vi "ngi get dataset secure.vi"(0 "ID":u16, 1 "Downloaded dataset":T4(array[cluster]), 3 "num sensor":i32[](array[numeric]), 4 "last packet type":u8[](array[numeric]), 5 "error in (no error)":errorcluster, 6 "State":u16(ring) items=["Init array", "Send get", "recive data", "abort secure download"], 7 "Node":i32=1, 8 "max download atempts":u8=10, 9 "download timeout":dbl=60.0 format="%#_13g", 10 "event_datadir":string, 12 "Recent events 2":T1(array[cluster]) {"SPS" format="%.1f"}, 13 "mac adresses":T3) -> (15 "Dataset":waveform(dbl)[][](array[waveform]), 16 "is downloading":bool[](array[boolean]), 18 "Safe Download":T2(array[cluster]), 19 "error out":errorcluster)   [LabVIEW 2017]
panel:
  out "busy?":bool[](array[boolean])
  out "channel mask":u8
  out "current time":timestamp
  out "dataset is complet":bool
  out "inserting data into array":bool
  out "last downloaded sample":u32
  out "num downloaded samples":u32
  out "dataset transfer completed":bool
  out "num samples in packet":i32
  out "Array":i32[][][](array[numeric])
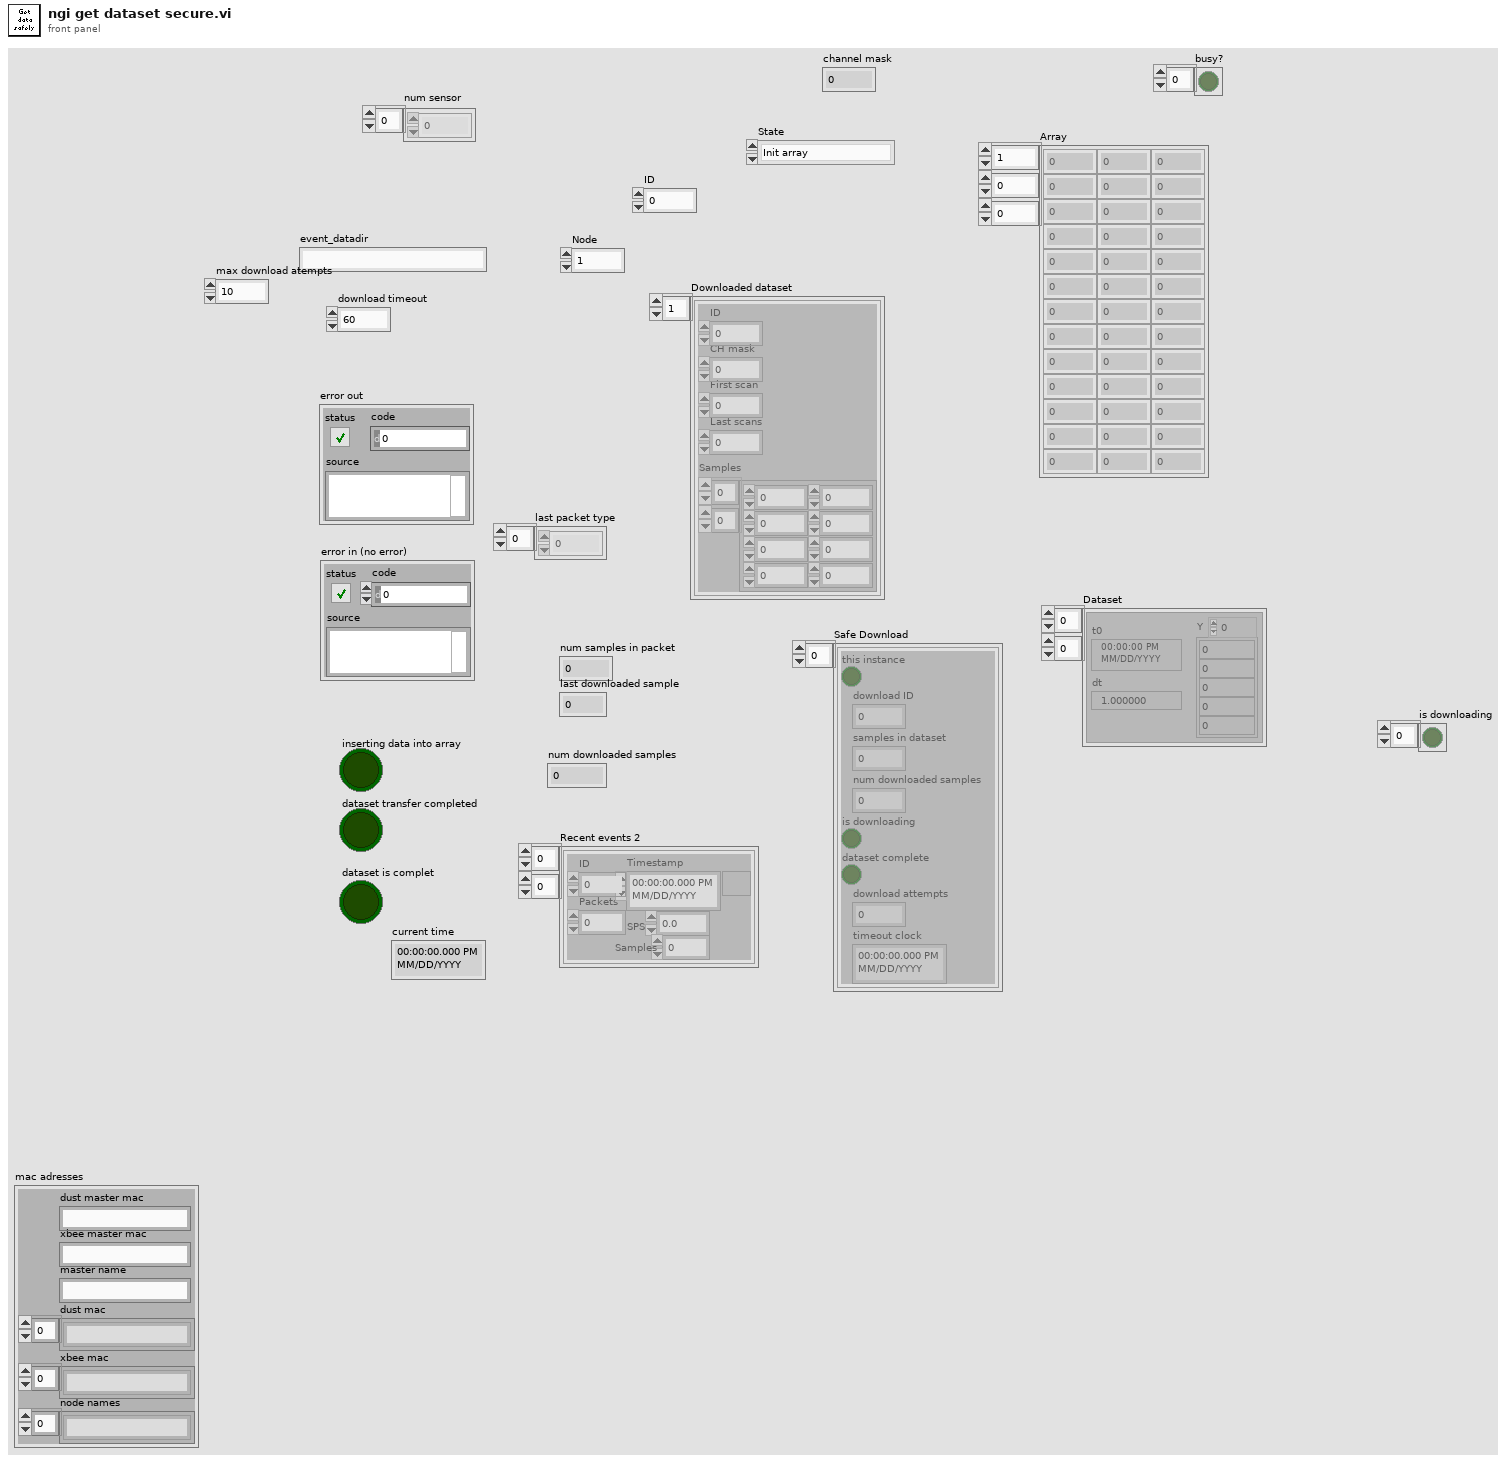
[diagram p1: front panel]
types:
  T1 = cluster{"ID":u16, "Timestamp":timestamp, "Packets":u16, "SPS":dbl, "Samples":u16}[][]
  T2 = cluster{"this instance":bool, "download ID":u32, "samples in dataset":u32, "num downloaded samples":u32, "is downloading":bool, "dataset complete":bool, "download attempts":u32, "timeout clock":timestamp}[]
  T3 = cluster{"dust master mac":string, "xbee master mac":string, "master name":string, "dust mac":string[], "xbee mac":string[], "node names":string[]}
  T4 = cluster{"ID":u16, "CH mask":u8, "First scan":u32, "Last scans":u32, "Samples":i32[][]}[]
  T5 = cluster{"this instance":bool, "download ID":u16, "samples in dataset":u32, "num downloaded samples":u32, "is downloading":bool, "dataset complete":bool, "download attempts":u32, "timeout clock":timestamp}
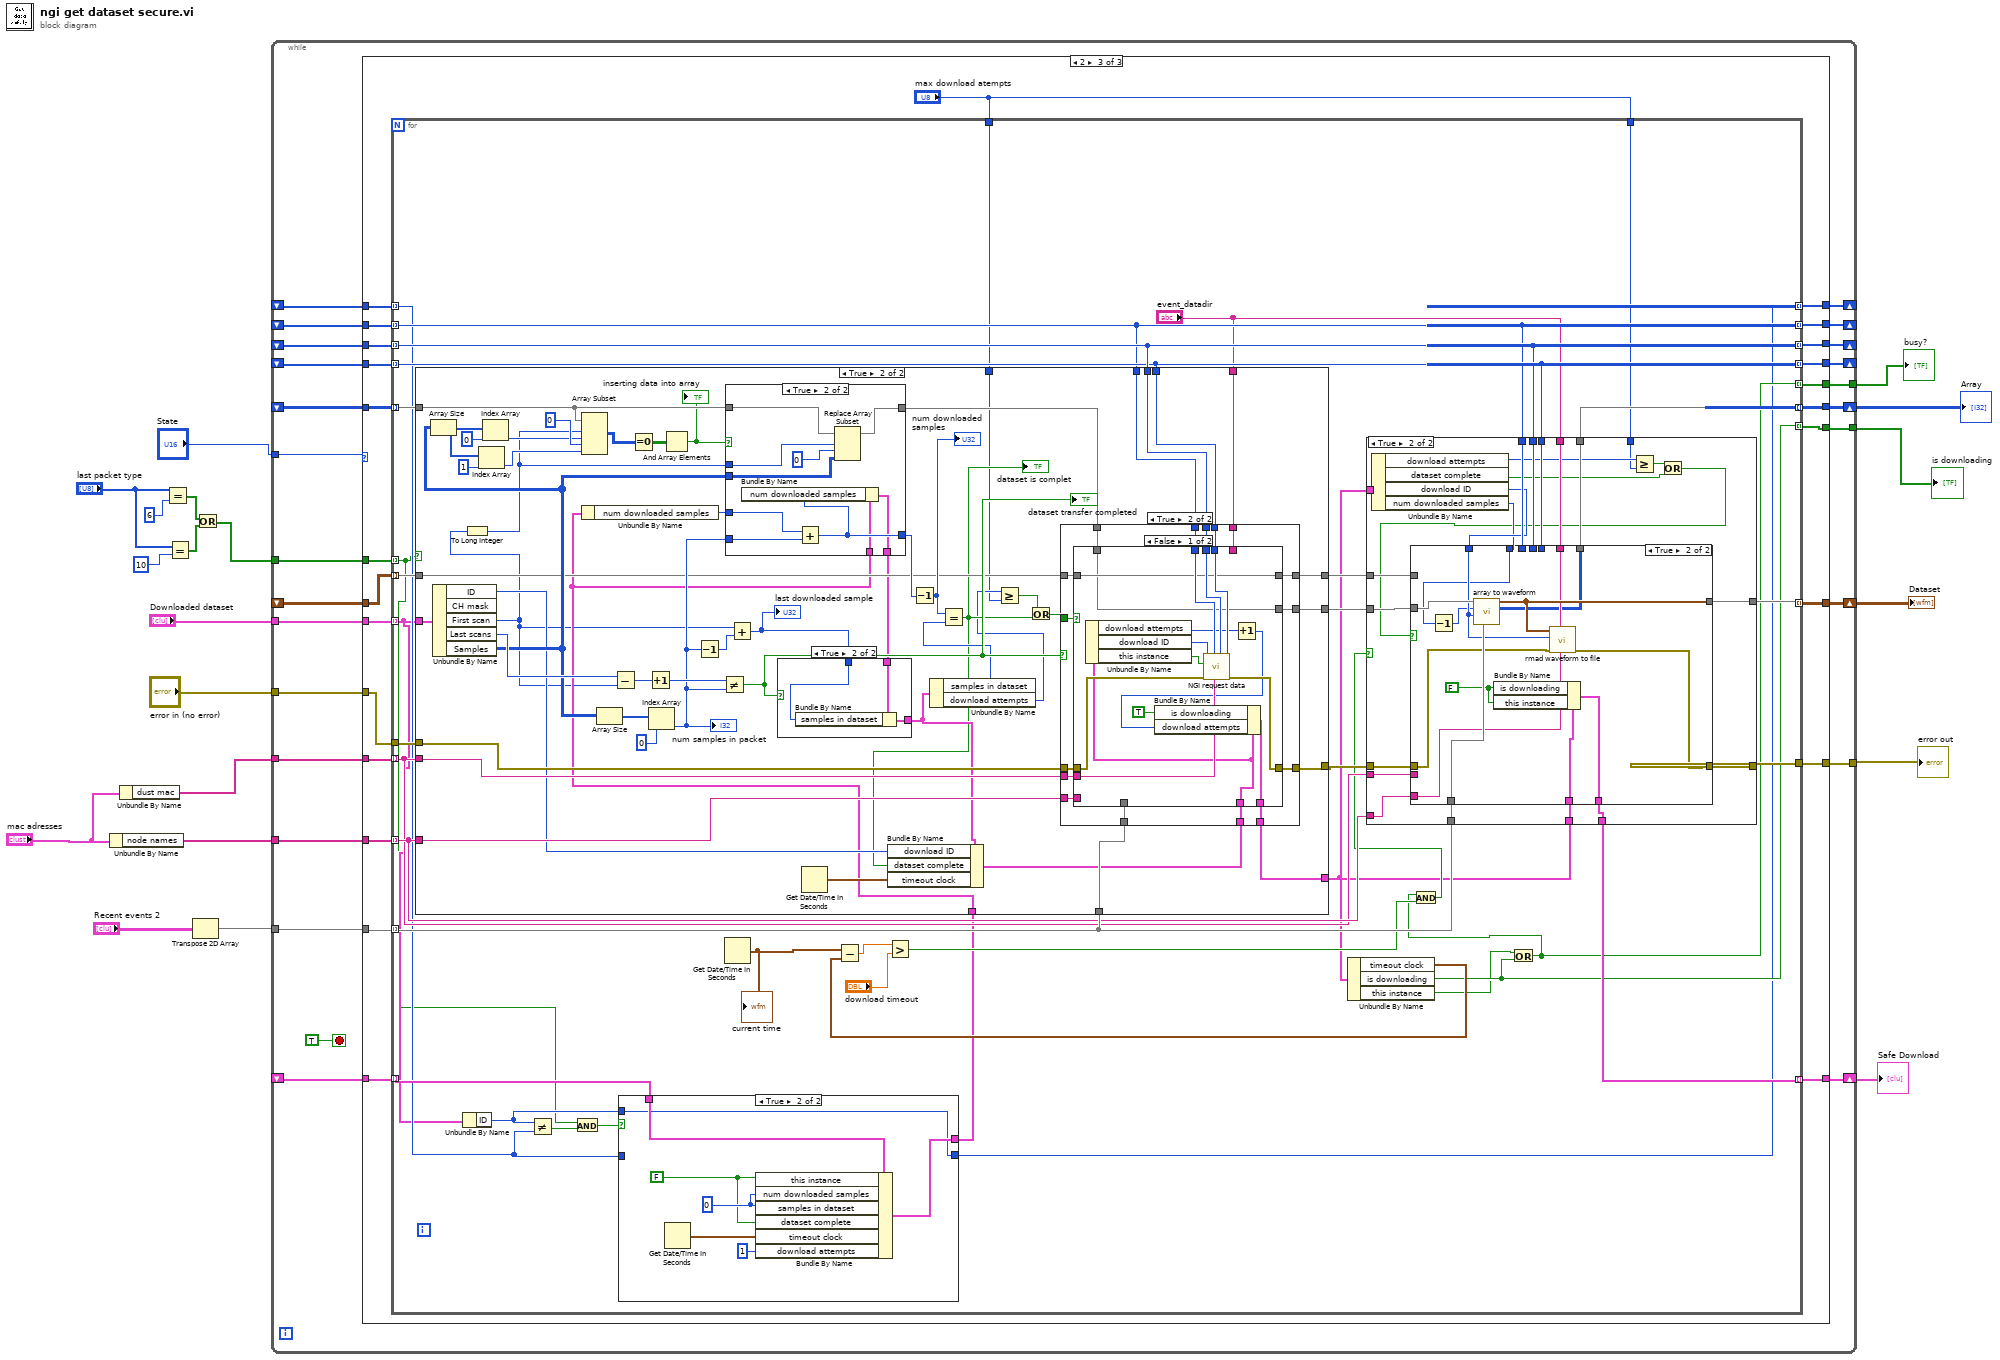
[diagram p0: block diagram]
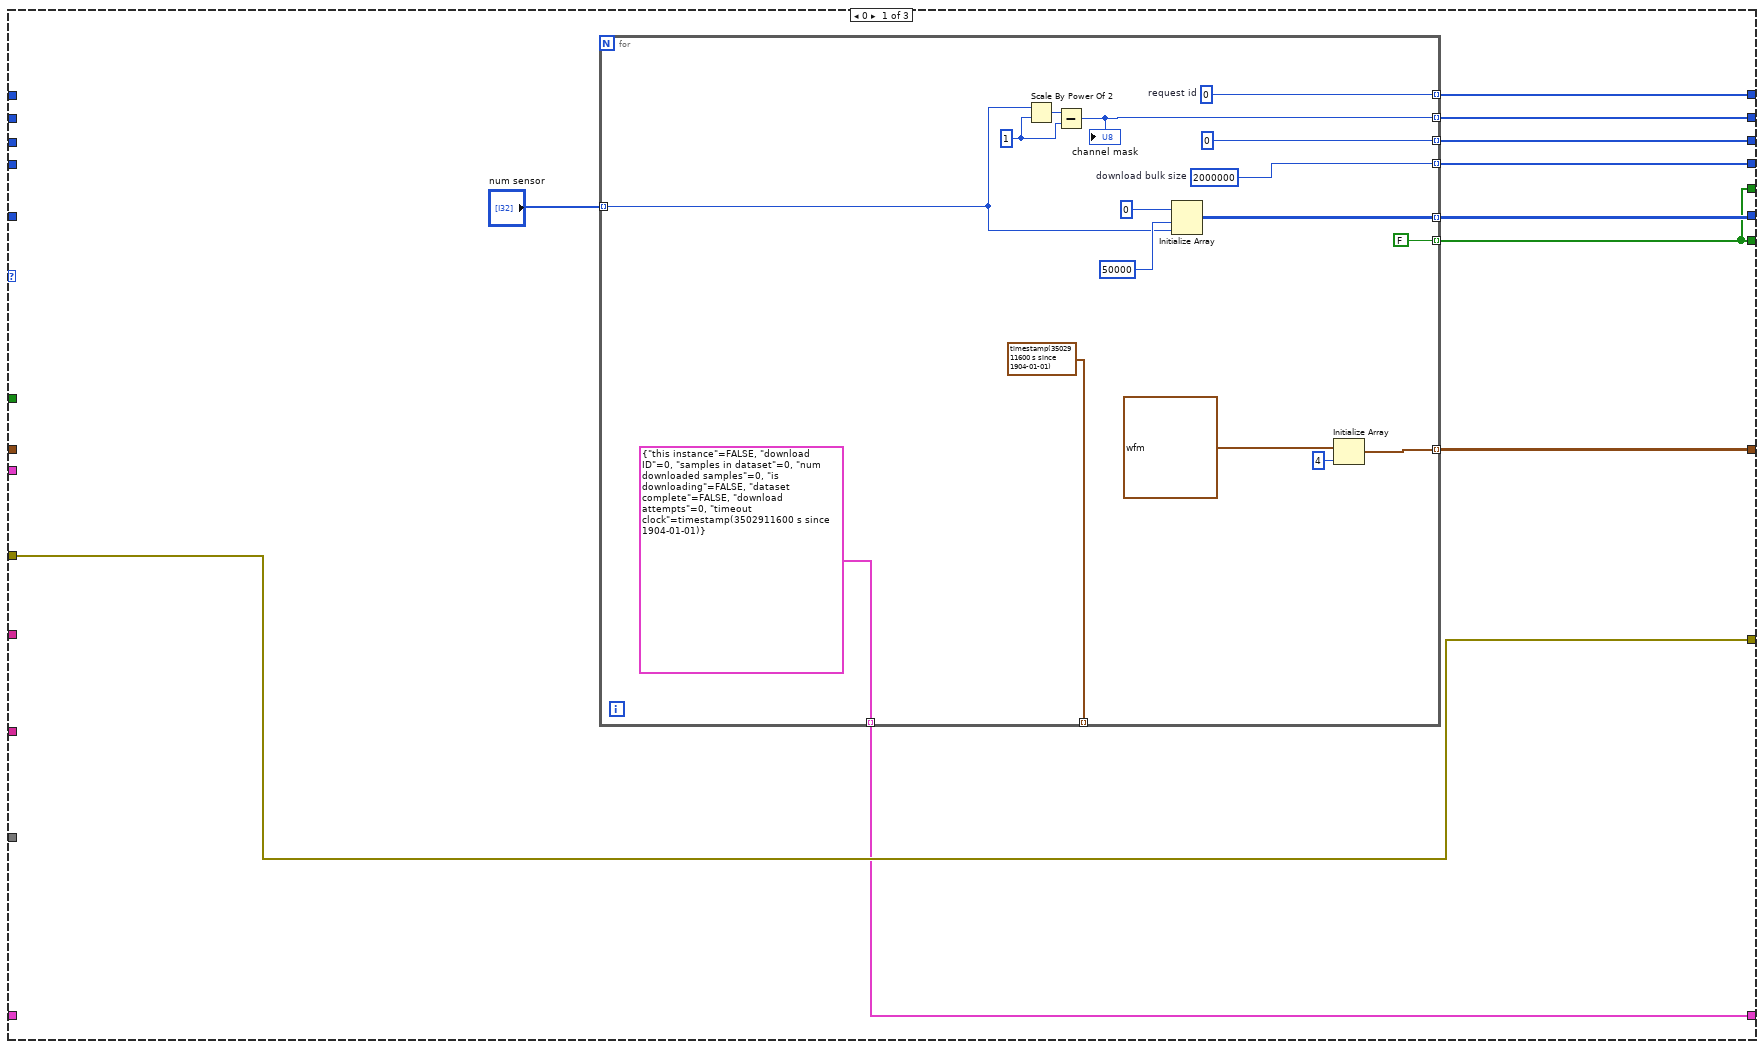
[diagram p2: hidden frame]
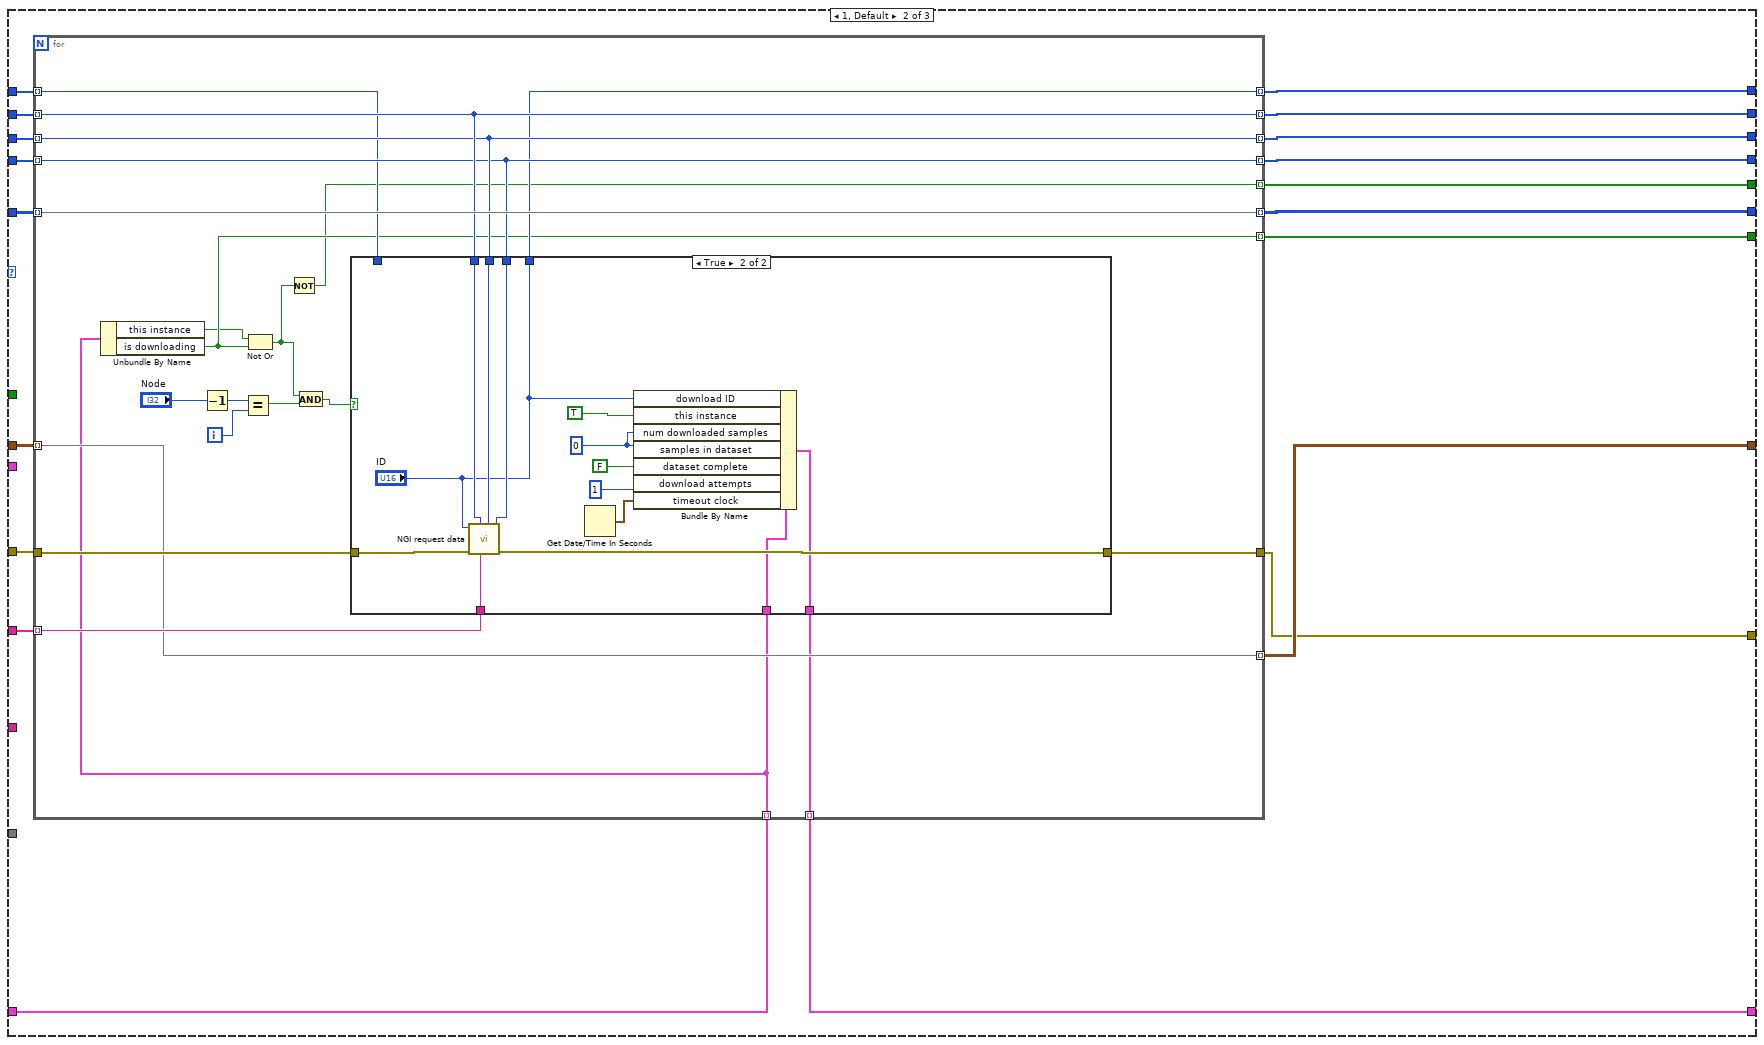
[diagram p3: hidden frame]
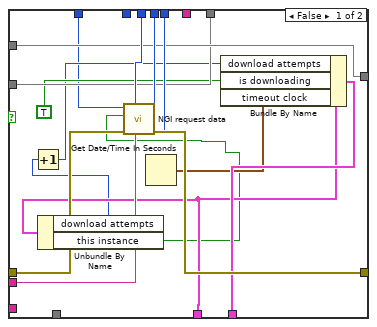
[diagram p7: hidden frame]
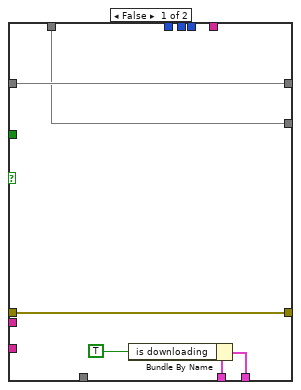
[diagram p9: hidden frame]
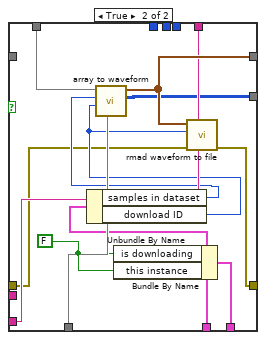
[diagram p10: hidden frame]
diagram:
  n1 = Unbundle By Name("mac adresses") -> ("node names"=w14:string[])
  n2 = Unbundle By Name("mac adresses") -> ("dust mac"=w11:string[])
  n3 = Equal?(x="last packet type", y=u8 6) -> (x = y?=w2:bool[])
  n4 = Equal?(x="last packet type", y=u8 10) -> (x = y?=w3:bool[])
  n5 = Transpose 2D Array(2D array="Recent events 2") -> (transposed array=w15:T1)
  n6 = Or(x=w2, y=w3) -> (x .or. y?=w1:bool[])
  n7 = while {
    tunnel: [w44] -> w10
    tunnel: "error in (no error)" -> [w43]
    tunnel: "State" -> [w31]
    tunnel: "Downloaded dataset" -> [w42]
    shift-right: [w25] -> w17
    shift-left: _ -> [w37]
    shift-right: [w38] -> _
    shift-left: _ -> [w33]
    shift-right: [w39] -> _
    shift-left: _ -> [w34]
    shift-right: [w40] -> _
    shift-left: _ -> [w35]
    shift-right: [w41] -> _
    shift-left: _ -> [w36]
    tunnel: w1 -> [w32]
    tunnel: w11 -> [w30]
    tunnel: w15 -> [w29]
    tunnel: w14 -> [w28]
    shift-right: [w27] -> w13
    shift-left: _ -> [w26]
    shift-right: [w24] -> w9
    shift-left: _ -> [w23]
    tunnel: [w22] -> w8
    tunnel: [w21] -> w6
    stop <- TRUE stop-if-true
    n8 = case shown="2" w31 {
      tunnel: [w49 w76 w134] -> w44
      tunnel: w43 -> [w49 w90 w141]
      tunnel: w42 -> [_ _ w152]
      tunnel: [w55 w81 w150] -> w25
      tunnel: [w54 w83 w143] -> w41
      tunnel: [w53 w85 w145] -> w40
      tunnel: [w52 w87 w147] -> w39
      tunnel: [w51 w89 w149] -> w38
      tunnel: w37 -> [_ w80 w151]
      tunnel: w36 -> [_ w82 w142]
      tunnel: w35 -> [_ w84 w144]
      tunnel: w34 -> [_ w86 w146]
      tunnel: w33 -> [_ w88 w148]
      tunnel: w32 -> [_ _ w140]
      tunnel: w30 -> [_ w79 w139]
      tunnel: w29 -> [_ _ w138]
      tunnel: w28 -> [_ _ w137]
      tunnel: [w50 w77 w135] -> w27
      tunnel: w26 -> [_ w78 w136]
      tunnel: [w48 w74 w132] -> w24
      tunnel: w23 -> [_ w75 w133]
      tunnel: [w46 w73 w131] -> w22
      tunnel: [w46 w72 w130] -> w21
      frame 0 {
        n9 = for {
          tunnel: [w70] -> w55 mode=indexing
          tunnel: [w63] -> w51 mode=indexing
          tunnel: [u32 0 ("element")] -> w53 mode=indexing
          tunnel: [w62] -> w54 mode=indexing
          tunnel: [w60] -> w52 mode=indexing
          tunnel: [timestamp(3502911600 s since 1904-01-01) ("seconds since 1Jan1904")] -> _ mode=indexing
          tunnel: [w64] -> w50 mode=indexing
          tunnel: [T5 {"this instance"=FALSE, "download ID"=0, "samples in dataset"=0, "num downloaded samples"=0, "is downloading"=FALSE, "dataset complete"=FALSE, "download attempts"=0, "timeout clock"=timestamp(3502911600 s since 1904-01-01)}] -> w48 mode=indexing
          tunnel: [FALSE] -> w46 mode=indexing
          tunnel: "num sensor" -> [w57] mode=indexing
          w62 = u32 2000000  # download bulk size
          w67 = u8 1 ("x")
          w63 = u16 0  # request id
          n10 = Scale By Power Of 2(n=w57, x=w67) -> (x*2^n=w68:u8)
          n11 = Subtract(x=w68, y=w67) -> (x-y=w60:u8)
          "channel mask" <- w60
          n12 = Initialize Array(0 ("element"), 50000 ("dimension size"), w57) -> (w70:i32[][])
          n13 = Initialize Array(waveform(dbl) {"t0"=timestamp(0 s since 1904-01-01), "dt"=1.0, "Y"=[]} ("Waveform"), 4 ("dimension size")) -> (w64:waveform(dbl)[])
        }
      }
      frame 1, Default {
        n14 = for {
          tunnel: [w101] -> w89 mode=indexing
          tunnel: w88 -> [w102] mode=indexing
          tunnel: [w105] -> w87 mode=indexing
          tunnel: w86 -> [w105] mode=indexing
          tunnel: [w104] -> w85 mode=indexing
          tunnel: w84 -> [w104] mode=indexing
          tunnel: [w103] -> w83 mode=indexing
          tunnel: w82 -> [w103] mode=indexing
          tunnel: [w108] -> w81 mode=indexing
          tunnel: w80 -> [w108] mode=indexing
          tunnel: w79 -> [w100] mode=indexing
          tunnel: w90 -> [w110]
          tunnel: [w111] -> w76
          tunnel: [w99] -> w77 mode=indexing
          tunnel: w78 -> [w99] mode=indexing
          tunnel: w75 -> [w97] mode=indexing
          tunnel: [w98] -> w74 mode=indexing
          tunnel: [w94] -> w73 mode=indexing
          tunnel: [w91] -> w72 mode=indexing
          i -> [w106]
          n15 = Unbundle By Name(w97) -> ("this instance"=w93:bool, "is downloading"=w94:bool)
          n16 = Decrement(x="Node") -> (x-1=w107:i32)
          n17 = Equal?(x=w107, y=w106) -> (x = y?=w96:bool)
          n18 = Not Or(1:w94, 2:w93) -> (0:w92:bool)
          n19 = Not(x=w92) -> (.not. x?=w91:bool)
          n20 = And(x=w92, y=w96) -> (x .and. y?=w95:bool)
          n21 = case shown="True" w95 {
            tunnel: [w114 w126] -> w111
            tunnel: w110 -> [w114 w127]
            tunnel: w105 -> [_ w125]
            tunnel: w104 -> [_ w124]
            tunnel: w103 -> [_ w123]
            tunnel: w102 -> [w113 _]
            tunnel: [w113 "ID"] -> w101
            tunnel: w100 -> [_ w128]
            tunnel: w97 -> [w112 w122]
            tunnel: [w112 w119] -> w98
            frame False {
            }
            frame True {
              w117 = u32 0 ("samples in dataset")
              n22 = call "NGI request data.vi"("stop"=w123, "start"=w124, "MAC source"=w128, "Channels"=w125, "error in (no error)"=w127, "ID"="ID") -> ("error out"=w126:errorcluster)  [unwired: 5 in]
              n23 = Get Date/Time In Seconds() -> (seconds since 1Jan1904=w121:timestamp)
              n24 = Bundle By Name(cluster=w122, "download ID"="ID", "this instance"=TRUE ("dataset complete"), "num downloaded samples"=w117, "samples in dataset"=w117, "dataset complete"=FALSE, "download attempts"=u32 1, "timeout clock"=w121) -> (w119:T5)
            }
          }
        }
      }
      frame 2 {
        n25 = for {
          tunnel: w152 -> [w157] mode=indexing
          tunnel: w151 -> [w190] mode=indexing
          tunnel: [w171] -> w150 mode=indexing
          tunnel: [w158] -> w149 mode=indexing
          tunnel: w148 -> [w159] mode=indexing
          tunnel: [w178] -> w147 mode=indexing
          tunnel: w146 -> [w178] mode=indexing
          tunnel: [w185] -> w145 mode=indexing
          tunnel: w144 -> [w185] mode=indexing
          tunnel: [w184] -> w143 mode=indexing
          tunnel: w142 -> [w184] mode=indexing
          tunnel: w141 -> [w187]
          tunnel: w140 -> [w153] mode=indexing
          tunnel: w139 -> [w181] mode=indexing
          tunnel: w138 -> [w183] mode=indexing
          tunnel: w137 -> [w182] mode=indexing
          tunnel: w136 -> [w186] mode=indexing
          tunnel: [w179] -> w135 mode=indexing
          tunnel: [w176] -> w134
          tunnel: w133 -> [w161] mode=indexing
          tunnel: [w170] -> w132 mode=indexing
          tunnel: [w167] -> w131 mode=indexing
          tunnel: [w165] -> w130 mode=indexing
          tunnel: "max download atempts" -> [w164]
          tunnel: "max download atempts" -> [w163]
          n26 = Unbundle By Name(w157) -> ("ID"=w156:u16)
          n27 = Not Equal?(x=w156, y=w159) -> (x != y?=w154:bool)
          n28 = And(x=w153, y=w154) -> (x .and. y?=w155:bool)
          n29 = case shown="True" w155 {
            tunnel: w161 -> [w192 w198]
            tunnel: [w192 w197] -> w160
            tunnel: [w191 w196] -> w158
            tunnel: w159 -> [w191 _]
            tunnel: w156 -> [_ w196]
            frame False {
            }
            frame True {
              w199 = u32 0 ("samples in dataset")
              w193 = FALSE ("dataset complete")
              n30 = Get Date/Time In Seconds() -> (seconds since 1Jan1904=w195:timestamp)
              n31 = Bundle By Name(cluster=w198, "this instance"=w193, "num downloaded samples"=w199, "samples in dataset"=w199, "dataset complete"=w193, "timeout clock"=w195, "download attempts"=u32 1) -> (w197:T5)
            }
          }
          n32 = case shown="True" w153 {
            tunnel: w157 -> [_ w312]
            tunnel: w190 -> [w258 w297]
            tunnel: w187 -> [w260 w290]
            tunnel: [w260 w289] -> w175
            tunnel: w181 -> [_ w288]
            tunnel: w178 -> [_ w287]
            tunnel: w185 -> [_ w286]
            tunnel: w184 -> [_ w285]
            tunnel: w183 -> [_ w283]
            tunnel: w182 -> [_ w282]
            tunnel: w186 -> [w259 w281]
            tunnel: [w259 w280] -> w180
            tunnel: "event_datadir" -> [_ w279]
            tunnel: [w258 w278] -> w172
            tunnel: w160 -> [w257 w269]
            tunnel: [w257 w276] -> w169
            tunnel: w163 -> [_ w261]
            frame False {
            }
            frame True {
              n33 = Unbundle By Name(w312) -> ("ID"=w275:u16, "First scan"=w267:u32, "Last scans"=w306:u32, "Samples"=w303:i32[][])  [unwired: 1 out]
              n34 = Array Size(array=w303) -> (size(s)=w301:i32[])
              n35 = To Long Integer(number=w267) -> (32bit integer=w266:i32)
              n36 = Index Array(array=w301, index=1) -> (element=w299:i32)
              n37 = Index Array(array=w301, index=0) -> (element=w300:i32)
              n38 = Array Subset(array=w297, index (row)=w266, length (row)=w300, index (col)=0 ("index"), length (col)=w299) -> (w296:i32[][])
              n39 = Unbundle By Name(w269) -> ("num downloaded samples"=w270:u32)
              n40 = Array Size(array=w303) -> (size(s)=w311:i32[])
              n41 = Subtract(x=w306, y=w267) -> (x-y=w309:u32)
              n42 = Equal To 0?(x=w296) -> (x = 0?=w298:bool[][])
              n43 = Increment(x=w309) -> (x+1=w308:u32)
              n44 = Index Array(array=w311, index=0) -> (element=w294:i32)
              "num samples in packet" <- w294
              n45 = And Array Elements(Boolean array=w298) -> (logical AND=w295:bool)
              "inserting data into array" <- w295
              n46 = Decrement(x=w294) -> (x-1=w307:i32)
              n47 = Not Equal?(x=w308, y=w294) -> (x != y?=w291:bool)
              "dataset transfer completed" <- w291
              n48 = case shown="True" w295 {
                tunnel: [w369 w378] -> w284
                tunnel: w266 -> [_ w377]
                tunnel: w303 -> [_ w376]
                tunnel: w297 -> [w369 w375]
                tunnel: w294 -> [_ w374]
                tunnel: [w367 w372] -> w293
                tunnel: w270 -> [w367 w373]
                tunnel: w269 -> [w368 w371]
                tunnel: [w368 w370] -> w268
                frame False {
                }
                frame True {
                  n49 = Add(x=w373, y=w374) -> (x+y=w372:u32)
                  n50 = Bundle By Name(cluster=w371, "num downloaded samples"=w372) -> (w370:T5)
                  n51 = Replace Array Subset(array=w375, new element=w376, index (row)=w377, index (col)=0 ("disabled index (col)")) -> (w378:i32[][])
                }
              }
              n52 = Add(x=w267, y=w307) -> (x+y=w274:u32)
              "last downloaded sample" <- w274
              n53 = case shown="True" w291 {
                tunnel: w274 -> [_ w366]
                tunnel: [w363 w365] -> w273
                tunnel: w268 -> [w363 w364]
                frame False {
                }
                frame True {
                  n54 = Bundle By Name(cluster=w364, "samples in dataset"=w366) -> (w365:T5)
                }
              }
              n55 = Get Date/Time In Seconds() -> (seconds since 1Jan1904=w277:timestamp)
              n56 = Decrement(x=w293) -> (x-1=w292:u32)
              "num downloaded samples" <- w292
              n57 = Unbundle By Name(w273) -> ("samples in dataset"=w271:u32, "download attempts"=w262:u32)
              n58 = Equal?(x=w292, y=w271) -> (x = y?=w263:bool)
              "dataset is complet" <- w263
              n59 = Bundle By Name(cluster=w273, "download ID"=w275, "dataset complete"=w263, "timeout clock"=w277) -> (w272:T5)
              n60 = Greater Or Equal?(x=w262, y=w261) -> (x >= y?=w265:bool)
              n61 = Or(x=w265, y=w263) -> (x .or. y?=w264:bool)
              n62 = case shown="True" w291 {
                tunnel: w264 -> [_ w334]
                tunnel: w290 -> [w318 w333]
                tunnel: [w318 w332] -> w289
                tunnel: w288 -> [_ w331]
                tunnel: w287 -> [_ w330]
                tunnel: w286 -> [_ w329]
                tunnel: w285 -> [_ w328]
                tunnel: w284 -> [w316 w327]
                tunnel: w283 -> [_ w326]
                tunnel: w282 -> [_ w325]
                tunnel: w281 -> [w317 w324]
                tunnel: [w317 w323] -> w280
                tunnel: w279 -> [_ w322]
                tunnel: [w316 w321] -> w278
                tunnel: w272 -> [w315 w320]
                tunnel: [w314 w319] -> w276
                frame False {
                  n63 = Bundle By Name(cluster=w315, "is downloading"=TRUE) -> (w314:T5)
                }
                frame True {
                  n64 = case shown="False" w334 {
                    tunnel: w333 -> [w349 w351]
                    tunnel: [w348 w350] -> w332
                    tunnel: w331 -> [w347 _]
                    tunnel: w330 -> [w346 _]
                    tunnel: w329 -> [w345 _]
                    tunnel: w328 -> [w344 _]
                    tunnel: w327 -> [w342 w362]
                    tunnel: w326 -> [_ w361]
                    tunnel: w325 -> [_ w359]
                    tunnel: w324 -> [w343 _]
                    tunnel: [w343 w360] -> w323
                    tunnel: w322 -> [_ w358]
                    tunnel: [w342 w357] -> w321
                    tunnel: w320 -> [w335 w356]
                    tunnel: [w341 w355] -> w319
                    frame False {
                      n65 = Unbundle By Name(w335) -> ("download attempts"=w340:u32, "download ID"=w337:u16, "this instance"=w336:bool)
                      n66 = call "NGI request data.vi"("stop"=w344, "start"=w345, "MAC source"=w347, "Channels"=w346, "error in (no error)"=w349, "this instance?"=w336, "ID"=w337) -> ("error out"=w348:errorcluster)  [unwired: 4 in]
                      n67 = Increment(x=w340) -> (x+1=w339:u32)
                      n68 = Bundle By Name(cluster=w335, "is downloading"=TRUE, "download attempts"=w339) -> (w341:T5)
                    }
                    frame True {
                      w352 = FALSE
                      n69 = Bundle By Name(cluster=w356, "is downloading"=w352, "this instance"=w352) -> (w355:T5)
                      n70 = Unbundle By Name(w355) -> ("samples in dataset"=w353:u32, "download ID"=w354:u16)
                      n71 = call "array to waveform.vi"("reset events"=w361, "dataset ID"=w354, "num samples in dataset"=w353, "array dataset"=w362) -> ("cleared array dataset out"=w357:i32[][], "waveform dataset"=w360:waveform(dbl)[])  [unwired: 6 in]
                      n72 = call "rmad waveform to file.vi"("node name"=w359, "event_datadir"=w358, "error in (no error)"=w351, "ID"=w354, "waveform dataset"=w360) -> ("error out"=w350:errorcluster)  [unwired: 6 in]
                    }
                  }
                }
              }
            }
          }
          n73 = Get Date/Time In Seconds() -> (seconds since 1Jan1904=w162:timestamp)
          "current time" <- w162
          n74 = Unbundle By Name(w169) -> ("timeout clock"=w168:timestamp, "is downloading"=w167:bool, "this instance"=w166:bool)
          n75 = Subtract(x=w162, y=w168) -> (x-y=w189:dbl)
          n76 = Greater?(x=w189, y="download timeout") -> (0:w174:bool)
          n77 = Or(x=w166, y=w167) -> (x .or. y?=w165:bool)
          n78 = And(x=w165, y=w174) -> (x .and. y?=w173:bool)
          n79 = case shown="True" w173 {
            tunnel: w175 -> [w203 w226]
            tunnel: [w203 w217] -> w176
            tunnel: w181 -> [_ w225]
            tunnel: w178 -> [_ w224]
            tunnel: w185 -> [_ w223]
            tunnel: w184 -> [_ w222]
            tunnel: w183 -> [_ w221]
            tunnel: w182 -> [_ w220]
            tunnel: w180 -> [w202 w219]
            tunnel: [w202 w218] -> w179
            tunnel: "event_datadir" -> [_ w216]
            tunnel: w172 -> [w201 w215]
            tunnel: [w201 w214] -> w171
            tunnel: w169 -> [w200 w213]
            tunnel: [w200 w212] -> w170
            tunnel: w169 -> [_ w211]
            tunnel: w164 -> [_ w204]
            frame False {
            }
            frame True {
              n80 = Unbundle By Name(w211) -> ("download attempts"=w208:u32, "dataset complete"=w206:bool, "download ID"=w210:u16, "num downloaded samples"=w209:u32)
              n81 = Greater Or Equal?(x=w208, y=w204) -> (x >= y?=w207:bool)
              n82 = Or(x=w207, y=w206) -> (x .or. y?=w205:bool)
              n83 = case shown="True" w205 {
                tunnel: w226 -> [w242 w244]
                tunnel: [w241 w243] -> w217
                tunnel: w225 -> [w240 _]
                tunnel: w224 -> [w239 _]
                tunnel: w223 -> [w238 _]
                tunnel: w222 -> [w237 _]
                tunnel: w221 -> [_ w256]
                tunnel: w220 -> [_ w254]
                tunnel: w219 -> [w236 _]
                tunnel: [w236 w255] -> w218
                tunnel: w216 -> [_ w253]
                tunnel: w215 -> [w235 w252]
                tunnel: [w235 w251] -> w214
                tunnel: w213 -> [w231 w250]
                tunnel: [w234 w249] -> w212
                tunnel: w210 -> [w228 w248]
                tunnel: w209 -> [_ w246]
                frame False {
                  n84 = Unbundle By Name(w231) -> ("download attempts"=w229:u32, "this instance"=w227:bool)
                  n85 = Increment(x=w229) -> (x+1=w230:u32)
                  n86 = call "NGI request data.vi"("stop"=w237, "start"=w238, "MAC source"=w240, "Channels"=w239, "error in (no error)"=w242, "this instance?"=w227, "ID"=w228) -> ("error out"=w241:errorcluster)  [unwired: 4 in]
                  n87 = Get Date/Time In Seconds() -> (seconds since 1Jan1904=w232:timestamp)
                  n88 = Bundle By Name(cluster=w231, "download attempts"=w230, "is downloading"=TRUE, "timeout clock"=w232) -> (w234:T5)
                }
                frame True {
                  w247 = FALSE
                  n89 = Decrement(x=w246) -> (x-1=w245:u32)
                  n90 = call "array to waveform.vi"("reset events"=w256, "dataset ID"=w248, "num samples in dataset"=w245, "array dataset"=w252) -> ("cleared array dataset out"=w251:i32[][], "waveform dataset"=w255:waveform(dbl)[])  [unwired: 6 in]
                  n91 = Bundle By Name(cluster=w250, "is downloading"=w247, "this instance"=w247) -> (w249:T5)
                  n92 = call "rmad waveform to file.vi"("node name"=w254, "event_datadir"=w253, "error in (no error)"=w244, "ID"=w248, "waveform dataset"=w255) -> ("error out"=w243:errorcluster)  [unwired: 6 in]
                }
              }
            }
          }
        }
      }
    }
  }
  "error out" <- w10
  "Array" <- w17
  "Dataset" <- w13
  "Safe Download" <- w9
  "is downloading" <- w8
  "busy?" <- w6
